vi "ROSE_FF_pdf.vi"() -> (5 "Plug in titles":string[](array[string]), 7 "Plug in values":string[](array[string]))   [LabVIEW 2010]
uses:
  Globals/Plug_in_data_global.vi
  Globals/Meas_global.vi
panel:
  out "FF 2":cluster{"Histogram of X":dbl[], "Axis":dbl[]}(graph)
  out "FF":cluster{"Histogram of X":dbl[], "Axis":dbl[]}(graph)
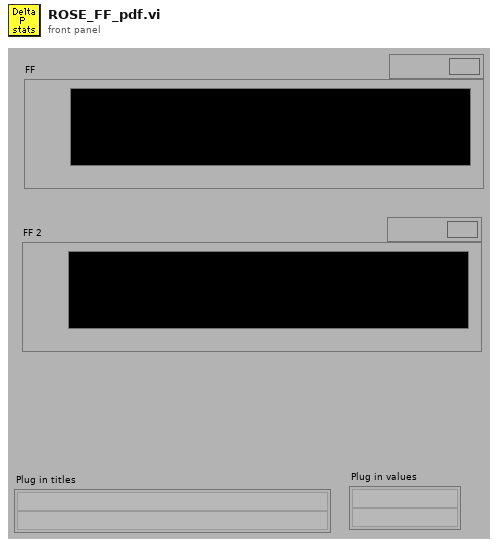
[diagram p1: front panel]
types:
  T1 = enum16{"Save no data", "Save data in new files", "Save data in existing files"}
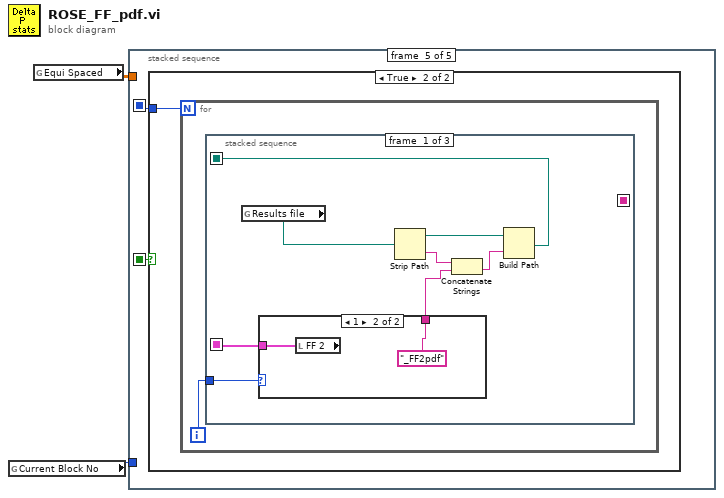
[diagram p0: block diagram]
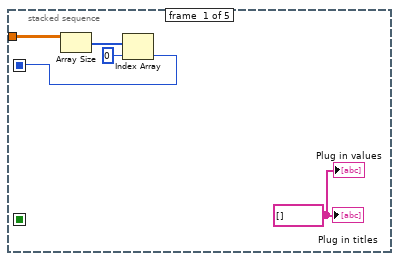
[diagram p2: hidden frame]
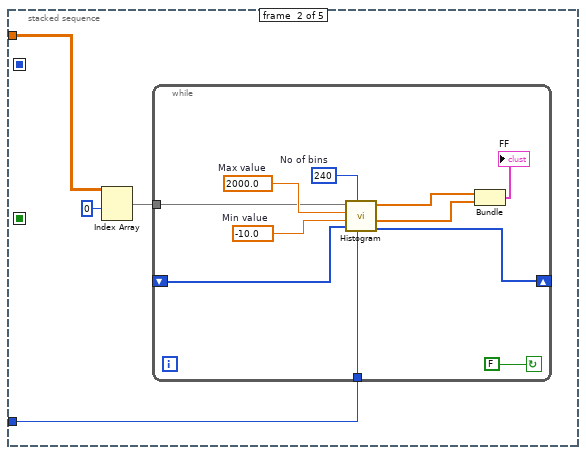
[diagram p3: hidden frame]
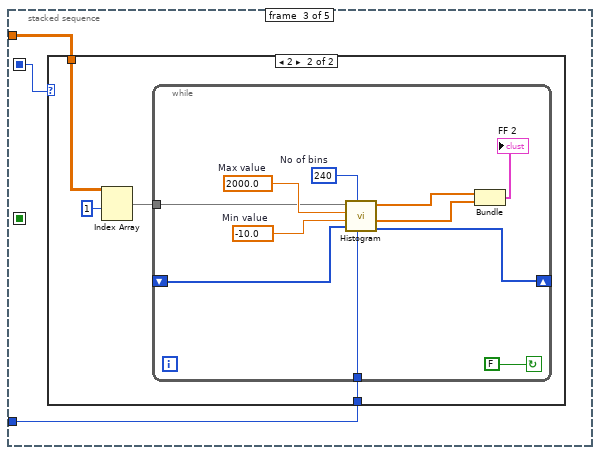
[diagram p4: hidden frame]
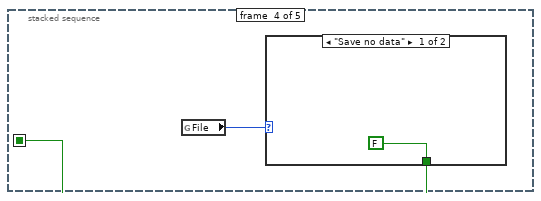
[diagram p6: hidden frame]
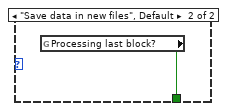
[diagram p7: hidden frame]
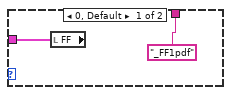
[diagram p9: hidden frame]
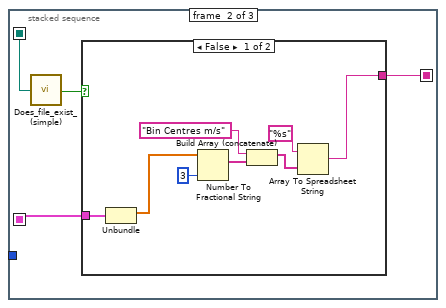
[diagram p10: hidden frame]
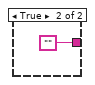
[diagram p11: hidden frame]
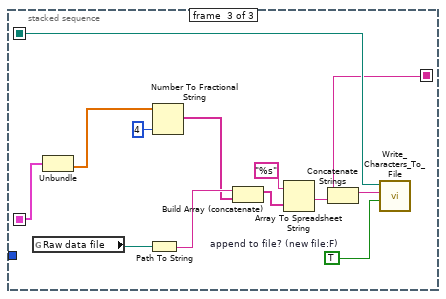
[diagram p12: hidden frame]
diagram:
  n1 = global read "Meas_global.vi" "Current Block No"() -> (w1:i32)
  n2 = global read "Plug_in_data_global.vi" "Equi Spaced"() -> (w2:dbl[][])
  n3 = stacked-sequence {
    seq-local: [_ _ _ w41 _] -> [_ _ _ _ w46]
    seq-local: [w3 _ _ _ _] -> [_ _ w23 _ w45]
    tunnel: w2 -> [w6 w9 w24 _ _]
    tunnel: w1 -> [_ w11 w25 _ _]
    frame #0 {
      w7 = string[] [] ("Plug in titles")
      n4 = Array Size(array=w6) -> (size(s)=w5:i32[])
      n5 = Index Array(array=w5, index=0 ("Index")) -> (element=w3:i32)
      "Plug in values" <- w7
      "Plug in titles" <- w7
    }
    frame #1 {
      n6 = Index Array(array=w9, index (row)=0) -> (element=w8:dbl[])  [unwired: 1 in]
      n7 = while {
        tunnel: w8 -> [w16]
        tunnel: w11 -> [w18]
        shift-left: _ -> [w17]
        shift-right: [w21] -> _
        stop <- FALSE continue-if-true
        w19 = 2000.0  # Max value
        w20 = -10.0  # Min value
        w22 = 240  # No of bins
        n8 = call "Histogram.vi"("Current Block No"=w18, "No of bins"=w22, "Shift Hist"=w17, "Min value"=w20, "Max value"=w19, "X"=w16) -> ("Shift Hist"=w21:i32[], "Histogram of X"=w14:dbl[], "Axis"=w15:dbl[])  [unwired: 1 in, 1 out]
        n9 = Bundle("Axis"=w15, "Histogram of X"=w14) -> (→"FF":cluster{"Axis":dbl[], "Histogram of X":dbl[]})  [unwired: 1 out]
      }
    }
    frame #2 {
      n10 = case shown="2" w23 {
        tunnel: w25 -> [_ w29]
        tunnel: w24 -> [_ w27]
        frame 0, Default {
        }
        frame 2 {
          n11 = Index Array(array=w27, index (row)=1) -> (element=w26:dbl[])  [unwired: 1 in]
          n12 = while {
            tunnel: w26 -> [w34]
            tunnel: w29 -> [w36]
            shift-left: _ -> [w35]
            shift-right: [w39] -> _
            stop <- FALSE continue-if-true
            w37 = 2000.0  # Max value
            w38 = -10.0  # Min value
            w40 = 240  # No of bins
            n13 = call "Histogram.vi"("Current Block No"=w36, "No of bins"=w40, "Shift Hist"=w35, "Min value"=w38, "Max value"=w37, "X"=w34) -> ("Shift Hist"=w39:i32[], "Histogram of X"=w32:dbl[], "Axis"=w33:dbl[])  [unwired: 1 in, 1 out]
            n14 = Bundle("Axis"=w33, "Histogram of X"=w32) -> (→"FF 2":cluster{"Axis":dbl[], "Histogram of X":dbl[]})  [unwired: 1 out]
          }
        }
      }
    }
    frame #3 {
      n15 = global read "Meas_global.vi" "File"() -> (w42:T1)
      n16 = case shown="\"Save no data\"" w42 {
        tunnel: [FALSE w44] -> w41
        frame "Save no data" {
        }
        frame "Save data in new files", Default {
          n17 = global read "Meas_global.vi" "Processing last block?"() -> (w44:bool)
        }
      }
    }
    frame #4 {
      n18 = case shown="True" w46 {
        tunnel: w45 -> [_ w47]
        frame False {
        }
        frame True {
          n19 = for {
            N: w47 -> [_]
            i -> [w48]
            n20 = stacked-sequence {
              seq-local: [w51 _ _] -> [_ w62 w79]
              seq-local: [w50 _ _] -> [_ w64 w78]
              seq-local: [_ w61 _] -> [_ _ w75]
              tunnel: w48 -> [w53 _ _]
              frame #0 {
                n21 = global read "Meas_global.vi" "Results file"() -> (w49:path)
                n22 = case shown="1" w53 {
                  tunnel: ["_FF1pdf" ("Substring") "_FF2pdf" ("Substring")] -> w52
                  tunnel: [w57 w59] -> w51
                  frame 0, Default {
                    n23 = local read "FF"() -> (w57:cluster{"Histogram of X":dbl[], "Axis":dbl[]})
                  }
                  frame 1 {
                    n24 = local read "FF 2"() -> (w59:cluster{"Histogram of X":dbl[], "Axis":dbl[]})
                  }
                }
                n25 = Strip Path(path=w49) -> (stripped path=w56:path, name=w55:string)
                n26 = Concatenate Strings(w55, w52) -> (w54:string)
                n27 = Build Path(base path=w56, name or relative path=w54) -> (appended path=w50:path)
              }
              frame #1 {
                n28 = call "Does_file_exist_(simple).vi"("Pathname"=w64) -> ("exists?"=w63:bool)
                n29 = case shown="False" w63 {
                  tunnel: w62 -> [w72 _]
                  tunnel: [w65 ""] -> w61
                  frame False {
                    n30 = Unbundle(w72) -> ("Histogram of X"=w70:dbl[])  [unwired: 1 out]
                    n31 = Number To Fractional String(number=w70, precision (6)=i16 3) -> (F-format string=w67:string[])  [unwired: 2 out]
                    n32 = Build Array (concatenate)("Bin Centres m/s" ("Input Element"), w67) -> (w69:string[])
                    n33 = Array To Spreadsheet String(array=w69, 3:"%s" ("format string")) -> (spreadsheet string=w65:string)  [unwired: 1 out]
                  }
                  frame True {
                  }
                }
              }
              frame #2 {
                w80 = TRUE  # append to file? (new file:F)
                n34 = global read "Meas_global.vi" "Raw data file"() -> (w85:path)
                n35 = Unbundle(w79) -> ("Axis"=w77:dbl[])  [unwired: 1 out]
                n36 = Path To String(path=w85) -> (string=w84:string)
                n37 = Number To Fractional String(number=w77, precision (6)=i16 4) -> (F-format string=w83:string[])  [unwired: 2 out]
                n38 = Build Array (concatenate)(w84, w83) -> (w82:string[])
                n39 = Array To Spreadsheet String(array=w82, 3:"%s" ("format string")) -> (spreadsheet string=w76:string)  [unwired: 1 out]
                n40 = Concatenate Strings(w75, w76) -> (w74:string)
                n41 = call "Write_Characters_To_File.vi"("file path (dialog if empty)"=w78, "character string"=w74, "append to file? (new file:F)"=w80) -> ()  [unwired: 2 in, 4 out]
              }
            }
          }
        }
      }
    }
  }
